vi "_FPGA_ReadyToStart.vi"(9 "Start_strobe_in":bool, 10 "Ready_latch_in":bool) -> (1 "Trigger_strobe_out":bool, 2 "Ready?":bool)   [LabVIEW 2018]
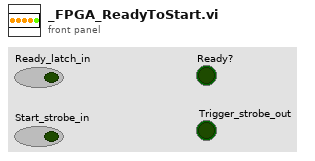
[diagram p1: front panel]
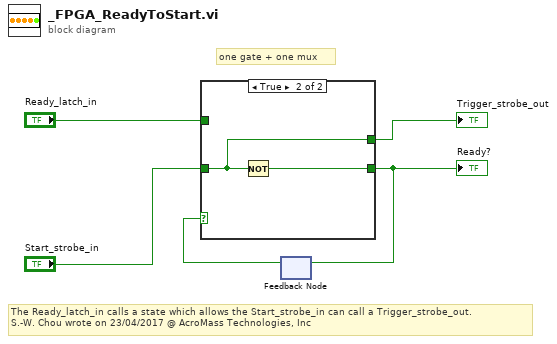
[diagram p0: block diagram]
diagram:
  # "one gate + one mux"
  # "The Ready_latch_in calls a state which allows the Start_strobe_in can call a Trigger_strobe_out.\nS.-W. Chou wrote on 23/04/2017 @ AcroMass Technologies, Inc"
  n1 = feedback #1() -> (w2:bool)  [unwired: 1 in]
  n2 = case shown="True" w2 {
    tunnel: "Ready_latch_in" -> [w6 _]
    tunnel: [w6 w8] -> w1
    tunnel: "Start_strobe_in" -> [_ w7]
    tunnel: [_ w7] -> w5
    frame False {
    }
    frame True {
      n3 = Not(x=w7) -> (.not. x?=w8:bool)
    }
  }
  "Trigger_strobe_out" <- w5
  "Ready?" <- w1
  n4 = feedback-in #1(w1) -> ()
